vi "AdquisicioDadesUSB.vi"(8 "Stop":refnum<vi>, 10 "user event":refnum<user-event>, 11 "AssaigActiu":refnum<vi>) -> ()   [LabVIEW 2017]
uses:
  <vilib>/DAQmx/read.llb/DAQmx Read (Analog 2D DBL NChan NSamp).vi
  <vilib>/DAQmx/miscellaneous.llb/DAQmx Fill In Error Info.vi
  <resource>/objmgr/daqmx.rc
panel:
  out "appended array":dbl[](array[numeric]) format="%#_8g"
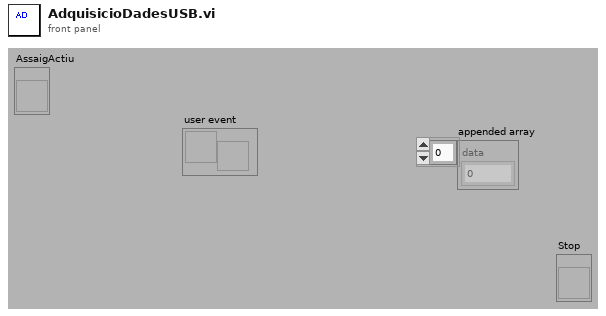
[diagram p1: front panel]
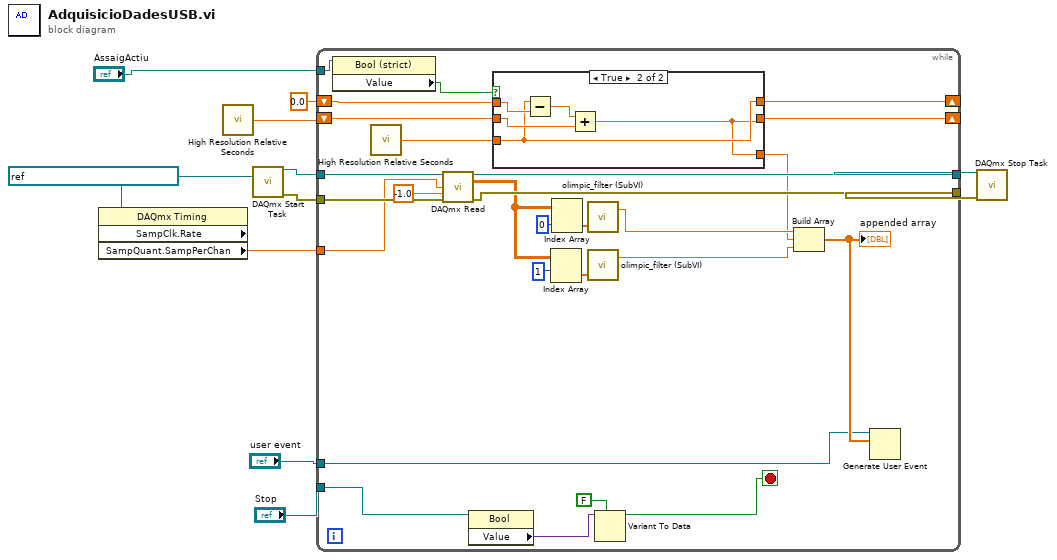
[diagram p0: block diagram]
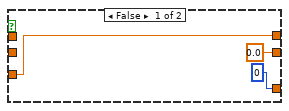
[diagram p2: hidden frame]
diagram:
  w5 = refnum<k21> "Esclatometre_USBAnalogIn" ("task/channels in")
  n1 = property class="DAQmx Timing" props=["SampClk.Rate", "SampQuant.SampPerChan"](reference=w5) -> ("SampQuant.SampPerChan"=w3:dbl)  [unwired: 1 in, 3 out]
  n2 = call <vilib>:"High Resolution Relative Seconds.vi"() -> ("relative seconds"=w2:dbl)
  n3 = call <vilib>:"DAQmx Start Task.vi"("task/channels in"=w5) -> ("task out"=w10:refnum<k21>, "error out"=w9:errorcluster)  [unwired: 13 in]
  n4 = while {
    tunnel: w10 -> [w28]
    tunnel: [w29] -> w11
    tunnel: w9 -> [w38]
    tunnel: "Stop" -> [w37]
    tunnel: [w34] -> w7
    tunnel: "user event" -> [w30]
    shift-right: [w20] -> _
    shift-left: w2 -> [w14]
    tunnel: "AssaigActiu" -> [w22]
    tunnel: w3 -> [w16]
    shift-right: [w13] -> _
    shift-left: 0.0 ("relative seconds") -> [w12]
    stop <- w33 stop-if-true
    n5 = property class="Bool (strict)"(reference=w22) -> ("Value"=w18:bool)  [unwired: 1 in, 2 out]
    n6 = call <vilib>:"High Resolution Relative Seconds.vi"() -> ("relative seconds"=w15:dbl)
    n7 = call-poly <vilib>:"DAQmx Read.vi"("task/channels in"=w28, "number of samples per channel"=w16, "timeout"=-1.0, "error in"=w38) -> ("task out"=w29:refnum<k21>, "data"=w23:dbl[][], "error out"=w34:errorcluster)  [unwired: 9 in]
    n8 = property class="Bool"(reference=w37) -> ("Value"=w36:variant)  [unwired: 1 in, 2 out]
    n9 = case shown="True" w18 {
      tunnel: [0.0 ("relative seconds") w42] -> w20
      tunnel: w15 -> [w39 w43]
      tunnel: [u32 0 ("millisecond timer value") w42] -> w17
      tunnel: w14 -> [_ w44]
      tunnel: [w39 w43] -> w13
      tunnel: w12 -> [_ w46]
      frame False {
      }
      frame True {
        n10 = Subtract(x=w43, y=w46) -> (x-y=w45:dbl)
        n11 = Add(x=w45, y=w44) -> (x+y=w42:dbl)
      }
    }
    n12 = Index Array(array=w23, index (row)=1) -> (element=w21:dbl[])  [unwired: 1 in]
    n13 = Index Array(array=w23, index (row)=0) -> (element=w27:dbl[])  [unwired: 1 in]
    n14 = call "olimpic_filter (SubVI).vi"("array"=w27) -> ("olimpic_filter"=w24:dbl)  [unwired: 1 out]
    n15 = call "olimpic_filter (SubVI).vi"("array"=w21) -> ("olimpic_filter"=w19:dbl)  [unwired: 1 out]
    n16 = Variant To Data(type=FALSE, Variant=w36) -> (data=w33:bool)  [unwired: 1 in, 1 out]
    n17 = Build Array(w24, w17, w19) -> (w31:dbl[])
    "appended array" <- w31
    n18 = Generate User Event(user event=w30, event data cluster=w31) -> ()  [unwired: 2 in, 2 out]
  }
  n19 = call <vilib>:"DAQmx Stop Task.vi"("task/channels in"=w11, "error in"=w7) -> ()  [unwired: 12 in, 2 out]
